vi "Start.vi"(8 "Error In":errorcluster, 11 "object in":refnum<class "Fgen PXI.lvclass">) -> (0 "Error Out":errorcluster, 3 "object out":refnum<class "Fgen PXI.lvclass">)   [LabVIEW 2023, in "FGEN.lvlib" / "Fgen PXI.lvlib" / "Fgen PXI.lvclass"]
uses:
  Fgen PXI.lvclass
  Fgen PXI.lvclass/Fgen PXI.ctl
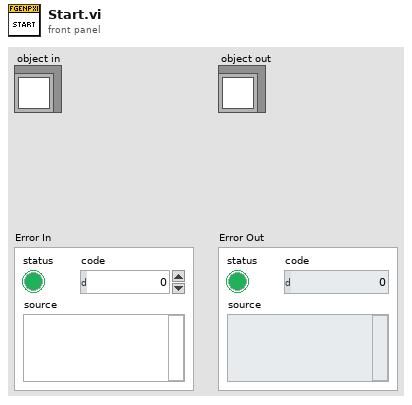
[diagram p1: front panel]
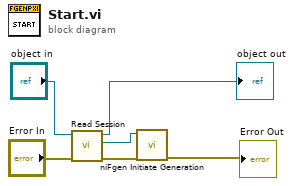
[diagram p0: block diagram]
diagram:
  n1 = call "Read Session.vi"("error in"="Error In", "Fgen PXI in"="object in") -> ("error out"=w4:errorcluster, "Session"=w3:refnum<k15>, "Fgen PXI out"=→"object out":refnum<class "Fgen PXI.lvclass">)  [unwired: 7 in]
  n2 = call <instrlib>:"niFgen Initiate Generation.vi"("error in (no error)"=w4, "Instrument Handle"=w3) -> ("error out"=→"Error Out":errorcluster)  [unwired: 8 in, 1 out]
